vi "Transmitter_Example  RxTx.vi"() -> ()   [LabVIEW 2022 SP3]
uses:
  <vilib>/imath/engines/lvmath/Plug In/_Char/NIMS_CH_character datatype.ctl
  <instrlib>/niUSRP/niUSRP Write Tx Data (CDB Cluster).vi
  <vilib>/imath/engines/lvmath2/RunTimeEngine/BuiltInFunctions/bitget/NIMS_bitget(SorV,SorV).vi
  <instcachedir>/0/NIMS_bitget(SorV,SorV)_FE8DB9DAC458464486262323321A5809.lvgen/NIMS_bitget(SorV,SorV)_FE8DB9DAC458464486262323321A5809_000.vi
  <vilib>/imathl/engines/lvmath/Functions/Error Handling/Create Error.vi
  <vilib>/imath/engines/lvmath2/RunTimeEngine/BuiltInFunctions/is_equal/NIMS_is_equal(GM).vi
  <instcachedir>/0/NIMS_is_equal(GM)_572A46D4183042F2BD2013DAF135E890.lvgen/NIMS_is_equal(GM)_572A46D4183042F2BD2013DAF135E890_001.vi
  <vilib>/imath/engines/lvmath2/RunTimeEngine/NodeEndStatement/NIMS_NodeEndStatement_Output.vi
  <instcachedir>/0/NIMS_NodeEndStatement_Output_53EC0D466D134D7ABD903AC30B43404B.lvgen/NIMS_NodeEndStatement_Output_53EC0D466D134D7ABD903AC30B43404B_010.vi
  <vilib>/imath/engines/lvmath2/RunTimeEngine/ErrorHandling/NIMS_Finalize Error.vi
panel:
  out "x = 0?":bool
  out "Led1":bool
  out "Led2":bool
  in  "String Non Critical Data 2":string="Critical Dataaaaa\nCritical Dataaaaa\nCritical Dataaaaa\nCritical Dataaaaa\nCritical Dataaaa§"
  in  "Modulation parameter 2":T1
  in  "stop 2":bool
  out "Waveform Graph":cluster{"t0":dbl, "dt":dbl, "Y":dbl[]}(graph)
  out "Frame Duration":dbl format="%#_6p"
  out "error out 2":errorcluster
  out "Bits length":i32
  out "Bits length 2":i32
  in  "String Non Critical Data":string="Critical Dataaaaa\nCritical Dataaaaa\nCritical Dataaaaa\nCritical Dataaaaa\nCritical Dataaaaa"
  in  "Alpha":dbl=0.05 min=0.0 max=1.0 step=0.05
  out "Frame Duration 2":dbl format="%#_6p"
  in  "New Non Critical Data":string="Critical Dataaaaa\nCritical Dataaaaa\nCritical Dataaaaa\nCritical Dataaaaa\nCritical Dataaaaa"
  in  "New Critical Data":string="Non Critical Data\nNon Critical Data\nNon Critical Data\nNon Critical Data\nNon Critical Data"
  out "AuxString":string
  out "AuxString 2":string
  in  "Previous Button":bool caption="Both Critical and Non Critical\nData must be equal size."
  in  "OFDM 4QAM / 16QAM":bool
  in  "String Critical Data":string="Non Critical Data\nNon Critical Data\nNon Critical Data\nNon Critical Data\nNon Critical Data"
  out "USRP CoercedParamters 2":T2={"coerced IQ rate"=100000.0, "coerced carrier frequency"=100000.0, "coerced gain"=0.0} {"coerced gain" format="%#_6f"; "coerced carrier frequency" format="%#_6p"; "coerced IQ rate" format="%#_6p"}
  in  "error in (no error) 2":errorcluster
  in  "USRP ControledParameters 2":T3={"active antenna"="TX1", "gain"=10.0, "carrier frequency"=2400000000.0, "IQ rate"=2000000.0} {"IQ rate" format="%#_6p"; "carrier frequency" format="%#_6p"; "gain" format="%#_6f"}
  in  "device names 2":refnum<k15>="RIO0"
  in  "stop 3":bool
  out "created new?":bool
  out "XY Graph":cdb[](graph)
  out "Modulation parameter":T1
  out "string 2":string
  out "SIG valid?":bool
  out "Frequency offset":dbl
  in  "stop":bool
  out "USRP CoercedParamters":T2={"coerced IQ rate"=100000.0, "coerced carrier frequency"=100000.0, "coerced gain"=0.0} {"coerced gain" format="%#_6f"; "coerced carrier frequency" format="%#_6p"; "coerced IQ rate" format="%#_6p"}
  out "error out":errorcluster
  in  "Trigger level":dbl=0.005 format="%f"
  in  "error in (no error)":errorcluster
  in  "USRP ControledParameters":T3={"active antenna"="RX1", "gain"=10.0, "carrier frequency"=2400000000.0, "IQ rate"=2000000.0} {"IQ rate" format="%#_6p"; "carrier frequency" format="%#_6p"; "gain" format="%#_6f"}
  in  "device names":refnum<k15>="RIO0"
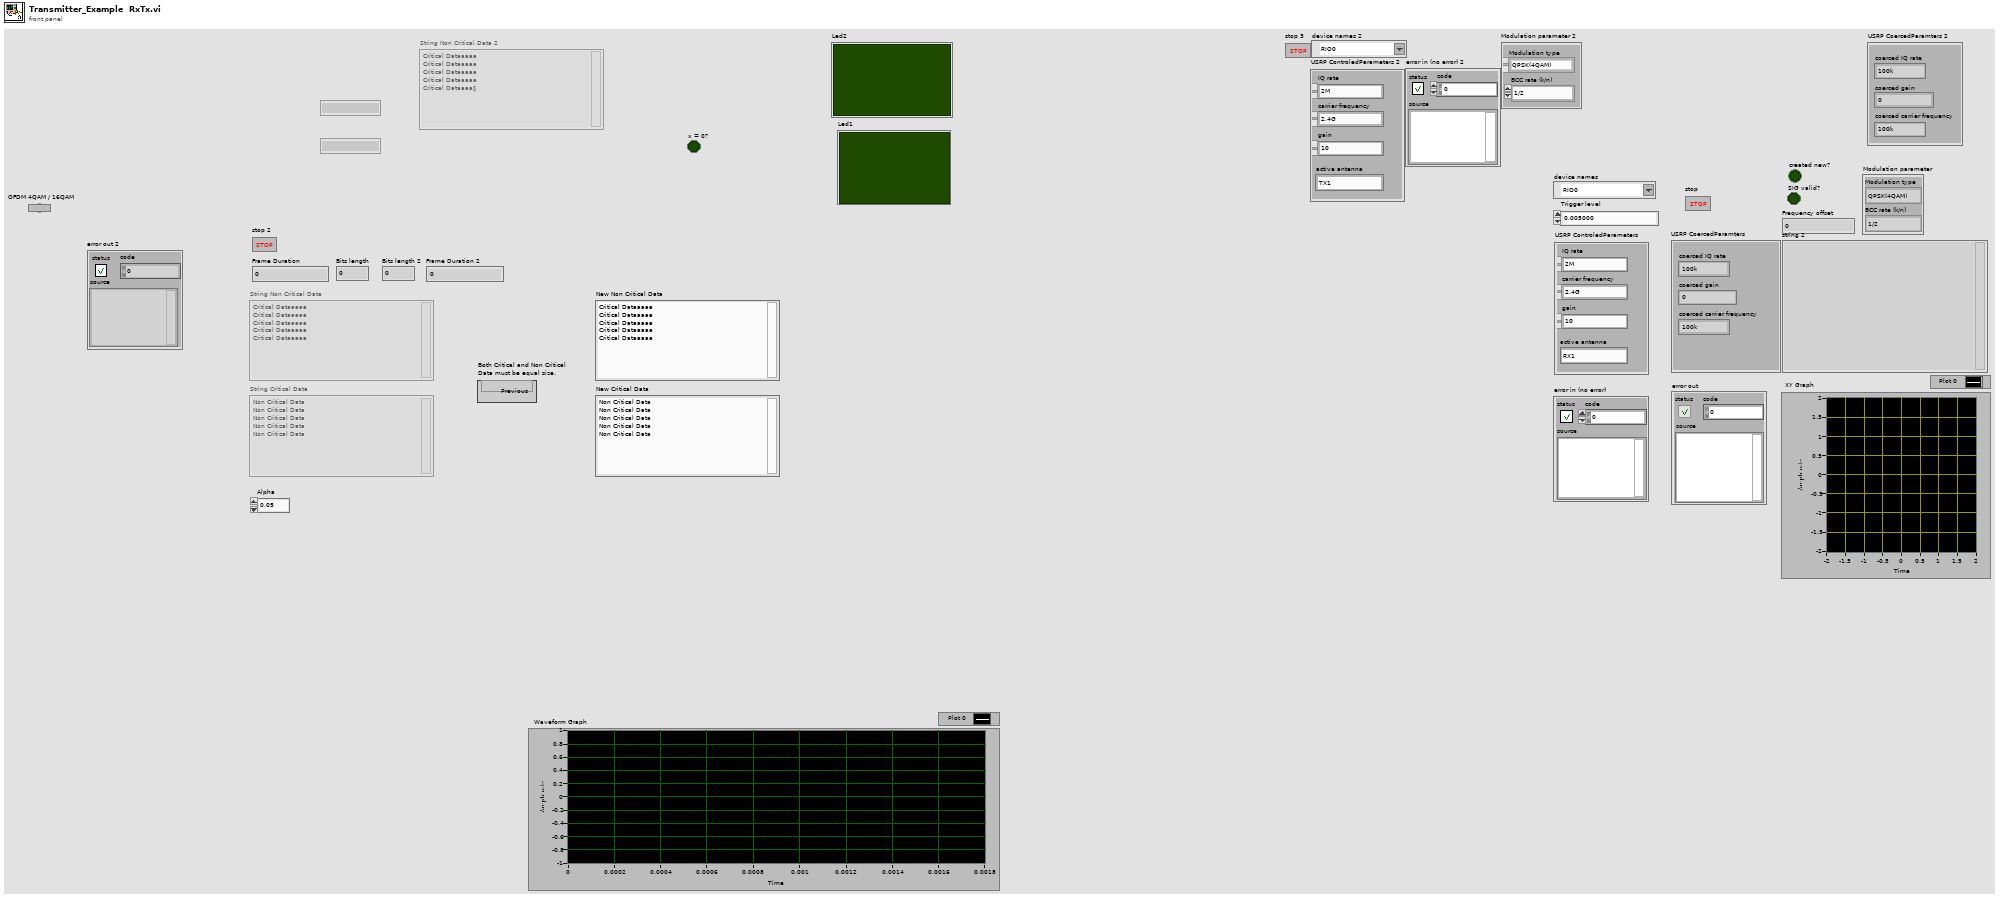
[diagram p1: front panel]
types:
  T1 = cluster{"Modulation type":enum16{"QPSK(4QAM)", "64QAM", "16QAM", "BPSK"}, "BCC rate (k/n)":enum16{"1/2", "2/3", "3/4"}}
  T2 = cluster{"coerced IQ rate":dbl, "coerced carrier frequency":dbl, "coerced gain":dbl}
  T3 = cluster{"active antenna":string, "gain":dbl, "carrier frequency":dbl, "IQ rate":dbl}
  T4 = typedef "NIMS_CH_character datatype.ctl" = cluster{"Numeric":u8}
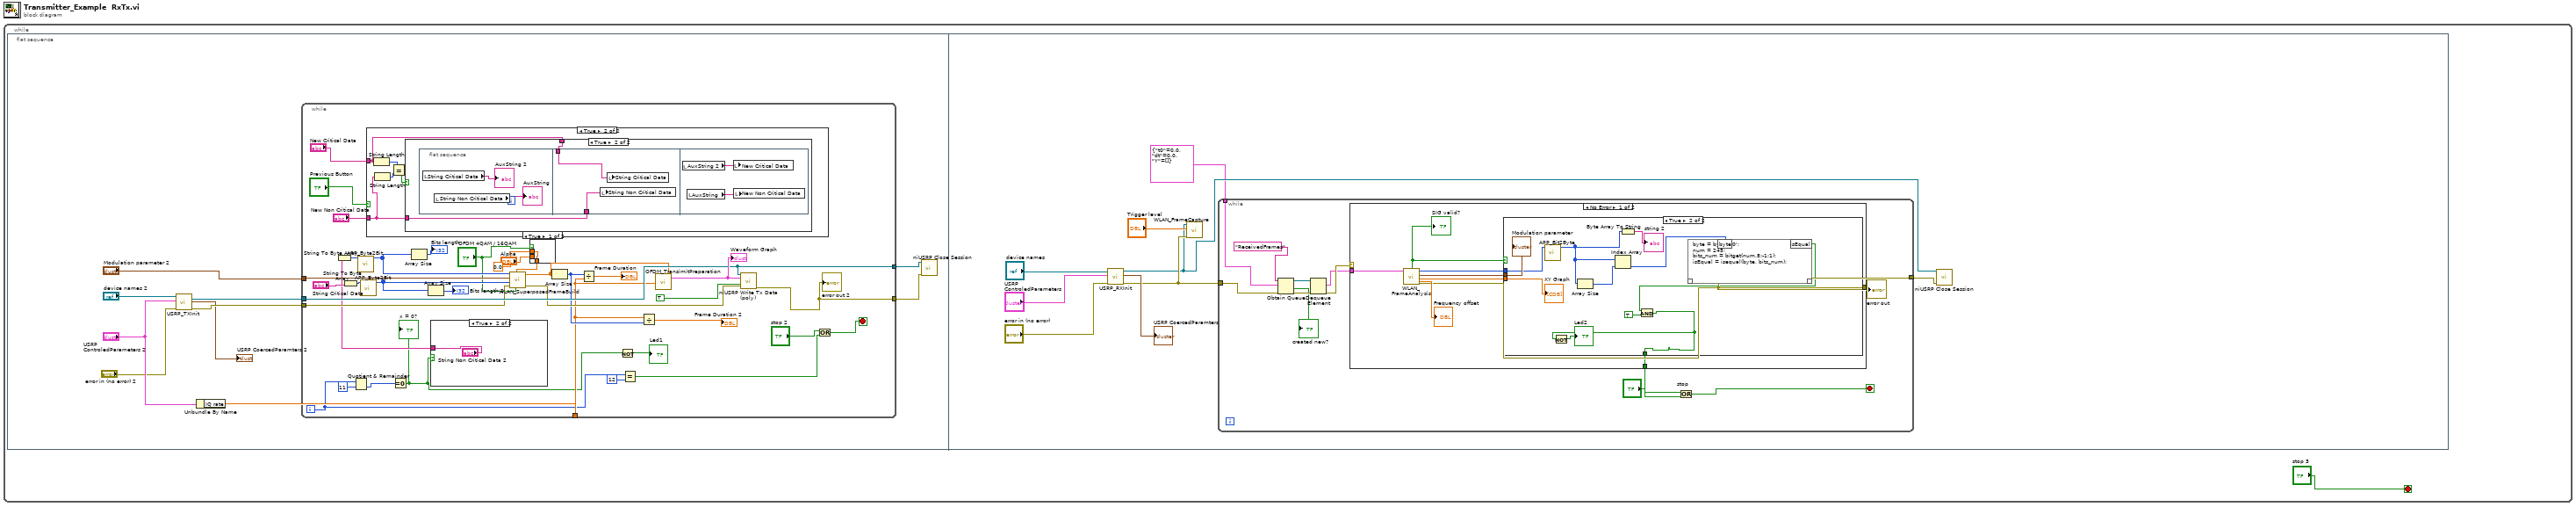
[diagram p0: block diagram]
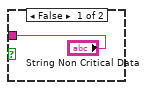
[diagram p2: hidden frame]
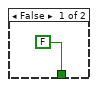
[diagram p6: hidden frame]
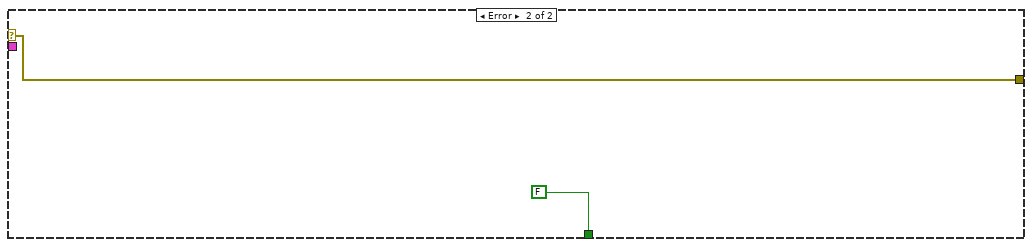
[diagram p7: hidden frame]
diagram:
  n1 = while {
    stop <- "stop 3" stop-if-true
    n2 = flat-sequence {
      frame #0 {
        n3 = call "USRP_TXInit.vi"("device names"="device names 2", "USRP ControledParameters"="USRP ControledParameters 2", "error in (no error)"="error in (no error) 2") -> ("session handle out"=w4:refnum<k15>, "USRP CoercedParamters"=→"USRP CoercedParamters 2":T2, "error out"=w8:errorcluster)  [unwired: 5 in]
        n4 = Unbundle By Name("USRP ControledParameters 2") -> ("IQ rate"=w11:dbl)
        n5 = while {
          tunnel: w4 -> [w43]
          tunnel: "Modulation parameter 2" -> [w37]
          tunnel: w8 -> [w36]
          tunnel: w11 -> [w31]
          tunnel: [w43] -> w9
          tunnel: [w42] -> w10
          i -> [w18]
          stop <- w21 stop-if-true
          n6 = String To Byte Array(string="String Critical Data") -> (unsigned byte array=w39:u8[])
          n7 = Quotient & Remainder(x=w18, y=11) -> (floor(x/y)=w19:i32)  [unwired: 1 out]
          n8 = call "APP_Byte2Bit.vi"("input byte stream"=w39) -> ("output bit stream"=w38:i8[])  [unwired: 10 in]
          n9 = case shown="True" "Previous Button" {
            tunnel: "New Non Critical Data" -> [_ w56]
            tunnel: "New Critical Data" -> [_ w52]
            frame False {
            }
            frame True {
              n10 = String Length(string=w52) -> (length=w55:i32)
              n11 = String Length(string=w56) -> (length=w54:i32)
              n12 = Equal?(x=w55, y=w54) -> (x = y?=w53:bool)
              n13 = case shown="True" w53 {
                tunnel: w56 -> [_ w58]
                tunnel: w52 -> [_ w57]
                frame False {
                }
                frame True {
                  n14 = flat-sequence {
                    tunnel: w58 -> [w62]
                    tunnel: w57 -> [w61]
                    frame #0 {
                      n15 = local read "String Critical Data"() -> (→"AuxString 2":string)
                      n16 = local read "String Non Critical Data"() -> (→"AuxString":string)
                    }
                    frame #1 {
                      n17 = local write "String Non Critical Data"(w62) -> ()
                      n18 = local write "String Critical Data"(w61) -> ()
                    }
                    frame #2 {
                      n19 = local read "AuxString 2"() -> (w63:string)
                      n20 = local read "AuxString"() -> (w64:string)
                      n21 = local write "New Critical Data"(w63) -> ()
                      n22 = local write "New Non Critical Data"(w64) -> ()
                    }
                  }
                }
              }
            }
          }
          n23 = Equal To 0?(x=w19) -> (x = 0?=w12:bool)
          "x = 0?" <- w12
          n24 = Array Size(array=w38) -> (size(s)=→"Bits length 2":i32)
          n25 = case shown="True" w12 {
            tunnel: ["String Non Critical Data" "String Non Critical Data 2"] -> w14
            frame False {
            }
            frame True {
            }
          }
          n26 = String To Byte Array(string=w14) -> (unsigned byte array=w40:u8[])
          n27 = call "APP_Byte2Bit.vi"("input byte stream"=w40) -> ("output bit stream"=w33:i8[])  [unwired: 10 in]
          n28 = Array Size(array=w33) -> (size(s)=→"Bits length":i32)
          n29 = case shown="True" "OFDM 4QAM / 16QAM" {
            tunnel: [w50 w51] -> w26
            tunnel: "Alpha" -> [_ w51]
            tunnel: 0.0 ("Alpha 2") -> [w50 _]
            frame True {
            }
            frame False {
            }
          }
          n30 = call "WLAN_SuperposedFrameBuild.vi"("OFDMON"="OFDM 4QAM / 16QAM", "Alpha"=w26, "error in (no error)"=w36, "data in 2"=w38, "Modulation parameter"=w37, "data in"=w33) -> ("error out"=w35:errorcluster, "output array"=w34:cdb[])  [unwired: 4 in]
          n31 = Array Size(array=w34) -> (size(s)=w32:i32)
          n32 = Divide(x=w32, y=w31) -> (x/y=→"Frame Duration":dbl)
          n33 = Not(x=w12) -> (.not. x?=→"Led1":bool)
          n34 = Equal?(x=w18, y=12) -> (x = y?=w16:bool)
          n35 = Divide(x=w31, y=w32) -> (x/y=→"Frame Duration 2":dbl)
          n36 = call "OFDM_TransimitPreparation.vi"("IQ rate"=w31, "array"=w34) -> ("output cluster"=w45:cluster{"t0":dbl, "dt":dbl, "Y":cdb[]})  [unwired: 9 in]
          "Waveform Graph" <- w45
          n37 = call-poly <instrlib>:"niUSRP Write Tx Data (poly).vi"("session handle"=w43, "data"=w45, "end of data?"=TRUE, "error in (no error)"=w35) -> ("error out"=w42:errorcluster)  [unwired: 10 in, 1 out]
          "error out 2" <- w42
          n38 = Or(x="stop 2", y=w16) -> (x .or. y?=w21:bool)
        }
        n39 = call <instrlib>:"niUSRP Close Session.vi"("session handle"=w9, "error in (no error)"=w10) -> ()  [unwired: 13 in, 1 out]
      }
      frame #1 {
        n40 = call "USRP_RXInit.vi"("device names"="device names", "USRP ControledParameters"="USRP ControledParameters", "error in (no error)"="error in (no error)") -> ("session handle out"=w66:refnum<k15>, "USRP CoercedParamters"=→"USRP CoercedParamters":T2, "error out"=w69:errorcluster)  [unwired: 5 in]
        n41 = call "WLAN_FrameCapture.vi"("error in (no error)"=w69, "Trigger level"="Trigger level", "session handle"=w66) -> ()  [unwired: 8 in]
        n42 = while {
          tunnel: w69 -> [w84]
          tunnel: cluster{"t0":dbl, "dt":dbl, "Y":cdb[]} {"t0"=0.0, "dt"=0.0, "Y"=[]} ("data") -> [w85]
          tunnel: [w77] -> w67
          stop <- w75 stop-if-true
          n43 = Obtain Queue(name (unnamed)="ReceivedFrames", element data type=w85, error in (no error)=w84) -> (queue out=w83:refnum<queue>, created new?=→"created new?":bool, error out=w80:errorcluster)  [unwired: 2 in]
          n44 = Dequeue Element(queue=w83, error in (no error)=w80) -> (element=w81:cluster{"t0":dbl, "dt":dbl, "Y":cdb[]}, error out=w82:errorcluster)  [unwired: 1 in, 2 out]
          n45 = case shown="No Error" w82 {
            selector: w82 -> [_ w165]
            tunnel: w81 -> [w87 _]
            tunnel: [w88 w165] -> w77
            tunnel: [w86 FALSE] -> w74
            frame No Error {
              n46 = call "WLAN_FrameAnalysis.vi"("input cluster"=w87) -> ("error out"=w88:errorcluster, "Constellation"=w90:cdb[], "Modulation parameter"=w89:T1, "output bits"=w91:i8[], "Frequency offset"=→"Frequency offset":dbl, "SIG valid?"=w92:bool)  [unwired: 5 in]
              "SIG valid?" <- w92
              n47 = case shown="True" w92 {
                tunnel: w91 -> [_ w102]
                tunnel: w90 -> [_ w104]
                tunnel: w89 -> [_ w105]
                tunnel: [FALSE w97] -> w86
                frame False {
                }
                frame True {
                  n48 = call "APP_Bit2Byte.vi"("input bit stream"=w102) -> ("output byte stream"=w101:u8[])  [unwired: 10 in]
                  n49 = Array Size(array=w101) -> (size(s)=w100:i32)
                  n50 = Index Array(array=w101, index=w100) -> (element=w98:u8)
                  n51 = Byte Array To String(unsigned byte array=w101) -> (string=→"string 2":string)
                  n52 = mathscript code="byte = byte - '0';\nnum = 245;\nbits_num = bitget(num,8:-1:1);\nisEqual = isequal(byte, bits_num);"("byte"=w98) -> ("isEqual"=w96:bool)  [unwired: 1 in, 1 out]
                  n53 = And(x=w96, y=TRUE) -> (x .and. y?=w97:bool)
                  n54 = Not(x=w97) -> (.not. x?=→"Led2":bool)
                  "Modulation parameter" <- w105
                  "XY Graph" <- w104
                }
              }
            }
            frame Error {
            }
          }
          "error out" <- w77
          n55 = Or(x="stop", y=w74) -> (x .or. y?=w75:bool)
        }
        n56 = call <instrlib>:"niUSRP Close Session.vi"("session handle"=w66, "error in (no error)"=w67) -> ()  [unwired: 13 in, 1 out]
      }
    }
  }
